vi "Easy Grid Setup.vi"(8 "error in":errorcluster, 9 "DataSource Data":string[][](array[string]), 10 "ColumnSetup":T1[](array[typedef]) {"MinWidth" min=2 step=1; "AutoSizeMode" items=["None"=1, "ColumnHeader"=2, "AllCellsExceptHeader"=4, "AllCells"=6, "DisplayedCellsExceptHeader"=8, "DisplayedCells"=10, "Fill"=16]; "FillWeight" min=1 max=100}, 11 ".net datagridview ref":refnum<k24>) -> (0 "error out":errorcluster, 1 "Grid RegisteredEvents":refnum<event-registration>, 2 "DataTable out":refnum<class "DataTable.lvclass">, 3 "DataGrid out":refnum<class "DataGridView.lvclass">)   [LabVIEW 2014]
doc: "Given a new datagridview .net container reference, this VI does all the sequencing and setup for your grid with a given input datasource table. It outputs the finished classes for datagrid and datatable, as well as the registered events for the grid that can be linked to an event structure for monitoring."
uses:
  System.Windows.Forms
  GridColumn/ColumnDefinition.ctl
  DataTable/DataTable.lvclass
  DataGridView/DataGridView.lvclass
  GridColumn/GridColumn.lvclass
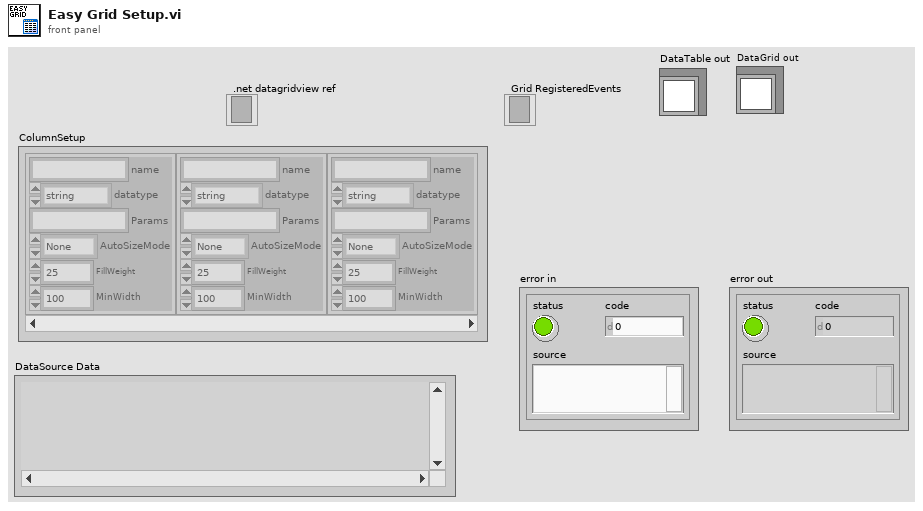
[diagram p1: front panel]
types:
  T1 = typedef "DataGrid.lvlib/GridColumn.lvclass/ColumnDefinition.ctl" = cluster{"name":string, "datatype":enum16{"string", "image", "check", "numeric", "timestamp", "button", "combo"}, "Params":string, "AutoSizeMode":i32, "FillWeight":sgl, "MinWidth":i32}
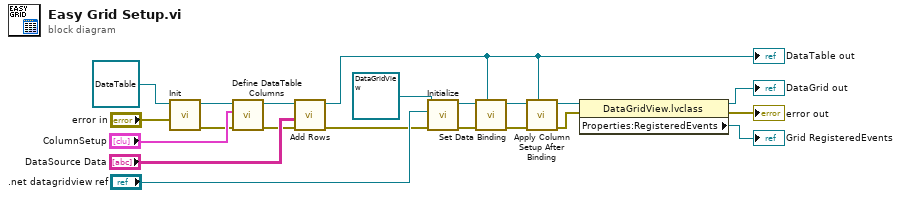
[diagram p0: block diagram]
diagram:
  n1 = call "Init.vi"("error in (no error)"="error in", "DataTable in"=refnum<class "DataTable.lvclass"> refnum) -> ("error out"=w5:errorcluster, "DataTable out"=w10:refnum<class "DataTable.lvclass">)  [unwired: 8 in]
  n2 = call "Define DataTable Columns.vi"("error in (no error)"=w5, "ColumnSetup"="ColumnSetup", "DataTable In"=w10) -> ("error out"=w3:errorcluster, "DataTable Out"=w9:refnum<class "DataTable.lvclass">)  [unwired: 7 in]
  n3 = call "Add Rows.vi"("error in (no error)"=w3, "String Data"="DataSource Data", "DataTable in"=w9) -> ("error out"=w6:errorcluster, "DataTable out"=w1:refnum<class "DataTable.lvclass">)  [unwired: 7 in]
  "DataTable out" <- w1
  n4 = call "Initialize.vi"("error in (no error)"=w6, "DataGridView"=".net datagridview ref", "DataGrid in"=refnum<class "DataGridView.lvclass"> refnum) -> ("error out"=w7:errorcluster, "DataGrid out"=w8:refnum<class "DataGridView.lvclass">)  [unwired: 7 in]
  n5 = call "Set Data Binding.vi"("DataTable Source"=w1, "error in (no error)"=w7, "DataGridView in"=w8) -> ("error out"=w15:errorcluster, "DataGridView out"=w17:refnum<class "DataGridView.lvclass">)  [unwired: 7 in]
  n6 = call "Apply Column Setup After Binding.vi"("DataTable"=w1, "error in (no error)"=w15, "DataGridView in"=w17) -> ("error out"=w20:errorcluster, "DataGridView out"=w2:refnum<class "DataGridView.lvclass">)  [unwired: 7 in]
  n7 = property class="DataGridView.lvclass"(reference=w2, error in=w20) -> (reference out=→"DataGrid out":refnum<class "DataGridView.lvclass">, error out=→"error out":errorcluster, "Properties:RegisteredEvents"=→"Grid RegisteredEvents":refnum<event-registration>)
